vi "触发拍照CCD1.vi"(8 "error in":errorcluster, 10 "Image Name":string="untitled", 11 "Session In":T2) -> (0 "error out":errorcluster, 1 "Buffer Number Out":u32, 2 "Image Out 3":T1(plugin-control), 3 "Session Out":T2)   [LabVIEW 2017]
uses:
  <vilib>/userdefined/High Color/IMAQdx.ctl
  <vilib>/vision/driver/NI_Vision_Acquisition_Software.lvlib
panel:
  out "TrgCnt out 2":i32
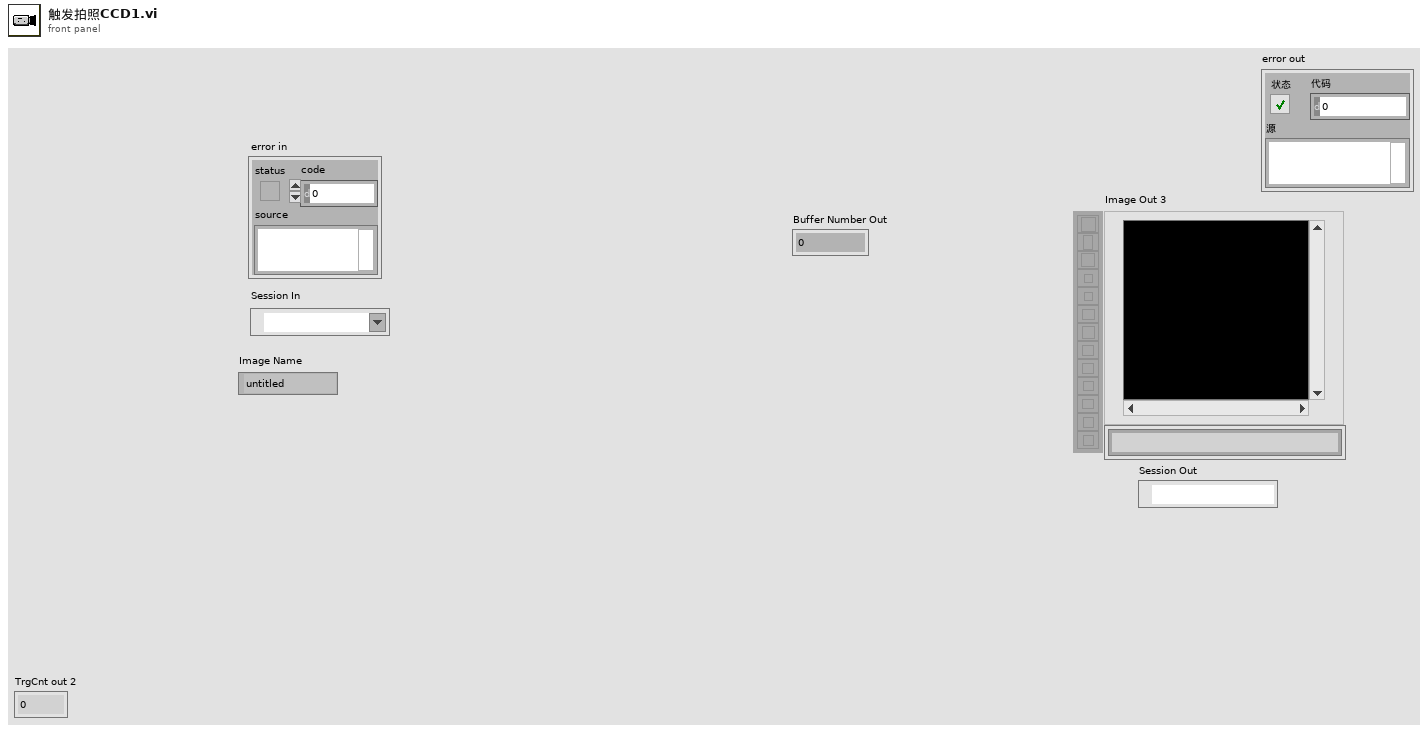
[diagram p1: front panel]
types:
  T1 = typedef "IMAQ Image.ctl" = refnum<image>
  T2 = typedef "IMAQdx.ctl" = refnum<k21>
  T3 = typedef "Image Type" = u32
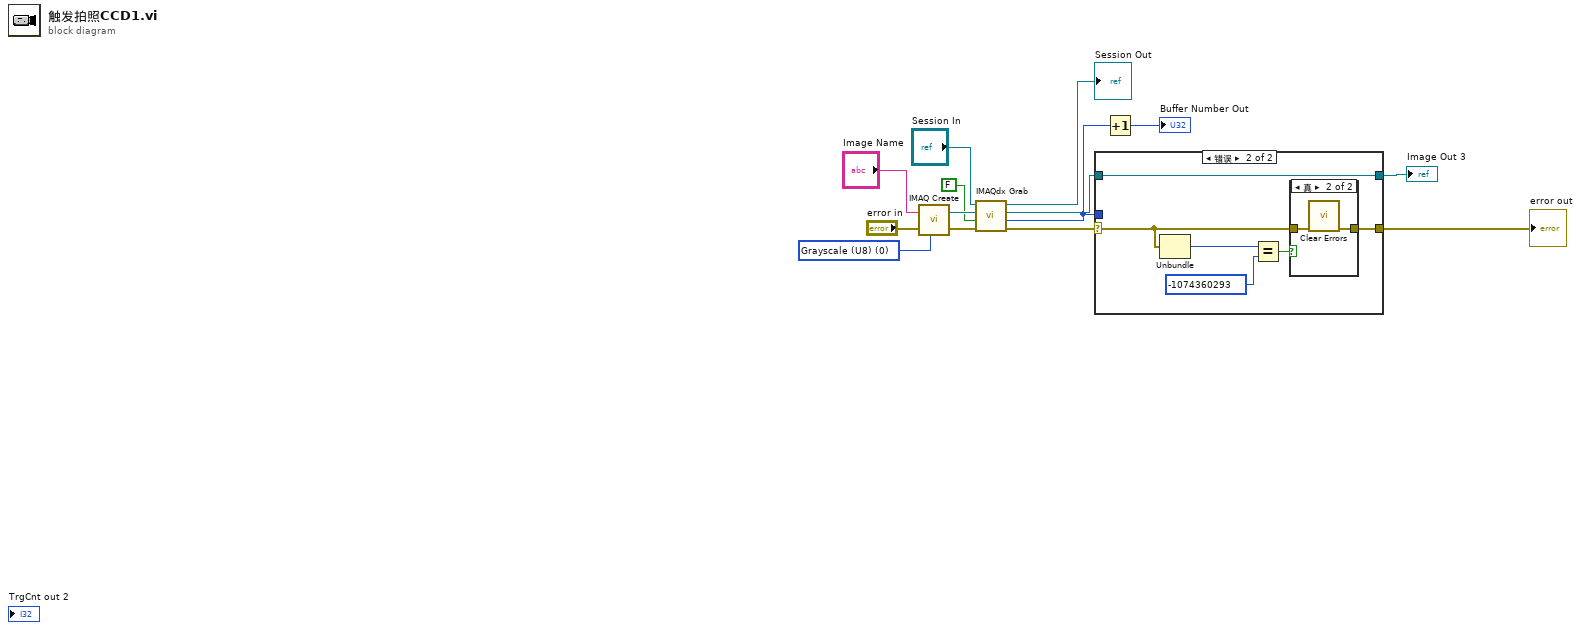
[diagram p0: block diagram]
diagram:
  w5 = T3 0 items=["Grayscale (U8)", "Grayscale (I16)", "Grayscale (SGL)", "Complex (CSG)", "RGB (U32)", "HSL (U32)", "RGB (U64)", "Grayscale (U16)"] ("Image Type")
  n1 = call "IMAQ Create"("Image Name"="Image Name", "Image Type"=w5, "error in (no error)"="error in") -> ("New Image"=w8:T1, "error out"=w9:errorcluster)  [unwired: 2 in]
  n2 = call <vilib>:"IMAQdx Grab.vi"("error in"=w9, "Wait for Next Buffer? (Yes)"=FALSE, "Image In"=w8, "Session In"="Session In") -> ("error out"=w13:errorcluster, "Buffer Number Out"=w6:u32, "Image Out"=w7:T1, "Session Out"=→"Session Out":T2)  [unwired: 4 in]
  n3 = case shown="错误" w13 {
    selector: w13 -> [w15 w22]
    tunnel: [w15 w21] -> w3
    tunnel: w7 -> [w16 w17]
    tunnel: [w16 w17] -> w2
    tunnel: w6 -> [_ _]
    frame No Error {
    }
    frame Error {
      n4 = Unbundle(w22) -> ("code"=w20:i32)  [unwired: 2 out]
      n5 = Equal?(x=w20, y=-1074360293) -> (x = y?=w19:bool)
      n6 = case shown="真" w19 {
        tunnel: w22 -> [w23 w25]
        tunnel: [w23 w24] -> w21
        frame False {
        }
        frame True {
          n7 = call <vilib>:"Clear Errors.vi"("error in (no error)"=w25) -> ("error out"=w24:errorcluster)  [unwired: 5 in, 1 out]
        }
      }
    }
  }
  "error out" <- w3
  "Image Out 3" <- w2
  n8 = Increment(x=w6) -> (x+1=→"Buffer Number Out":u32)
